vi "main.vi"() -> ()   [LabVIEW 2018]
uses:
  Ctrls/state.ctl
panel:
  out "Raw signal":u8[](graph)
  out "Output image":picture
  in  "Stop":bool
  in  "Save Image":bool
  in  "Image Name":string
  in  "Image upside down":bool
  out "Processing...":bool
  in  "Decode":bool
  in  "Input File":path
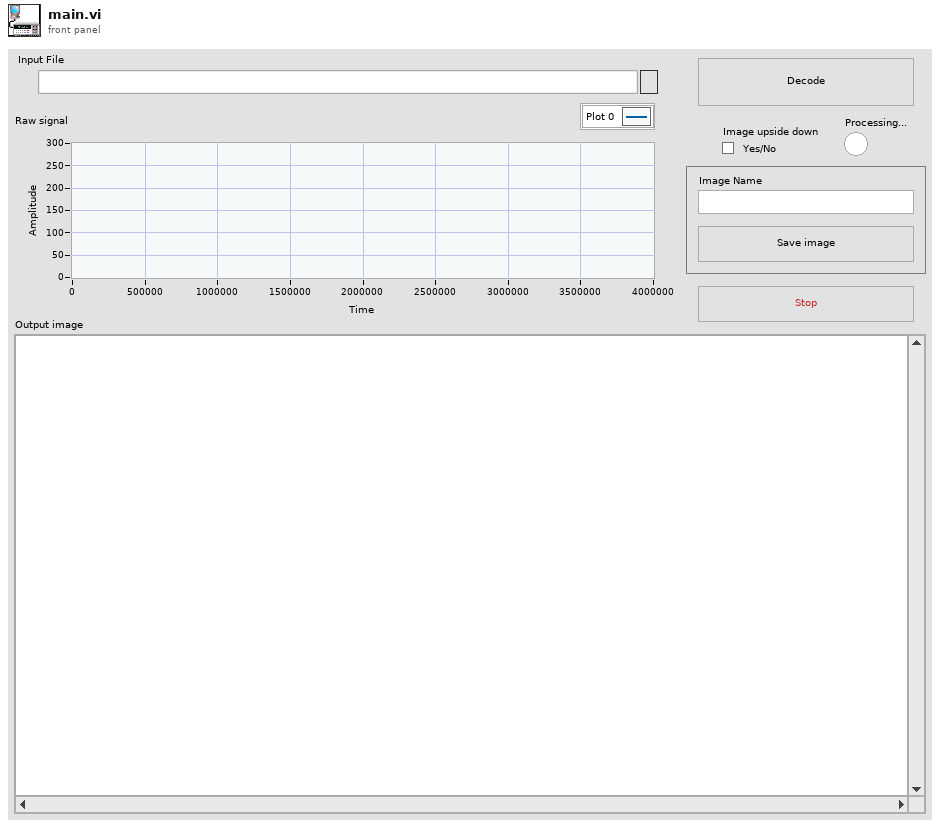
[diagram p1: front panel]
types:
  T1 = typedef "state.ctl" = enum16{"init", "decode", "quit", "UI", "save"}
  T2 = typedef "imagedata.ctl" = cluster{"image type":i32, "image depth":i32, "image":u8[], "mask":u8[], "colors":u32[], "Rectangle":cluster{"left":i16, "top":i16, "right":i16, "bottom":i16}}
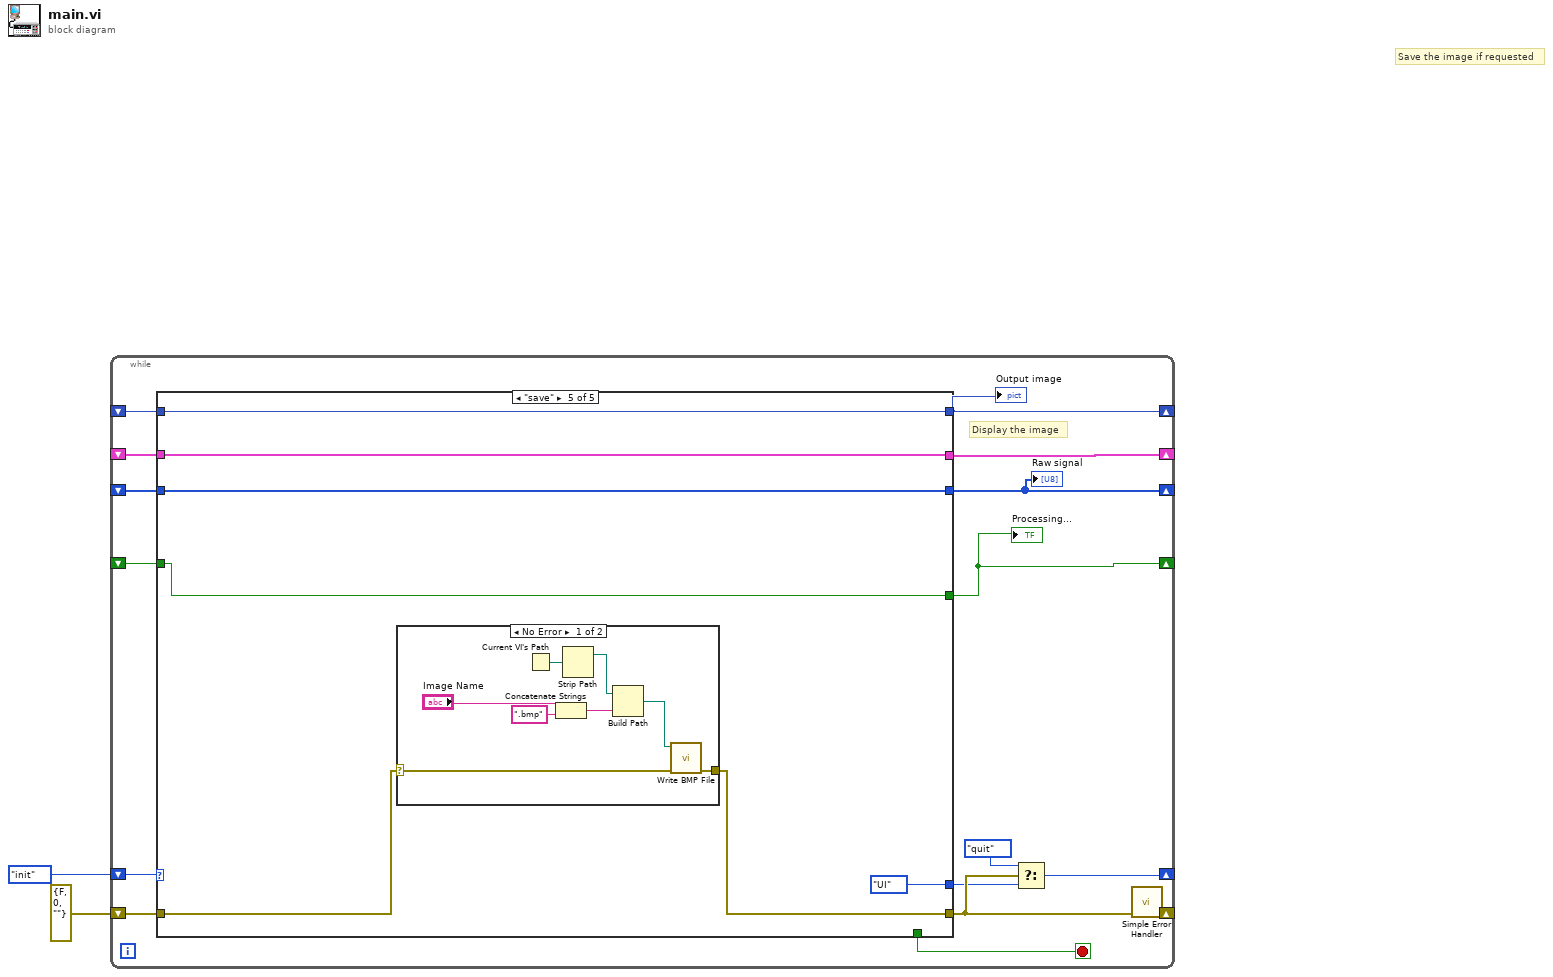
[diagram p0: block diagram]
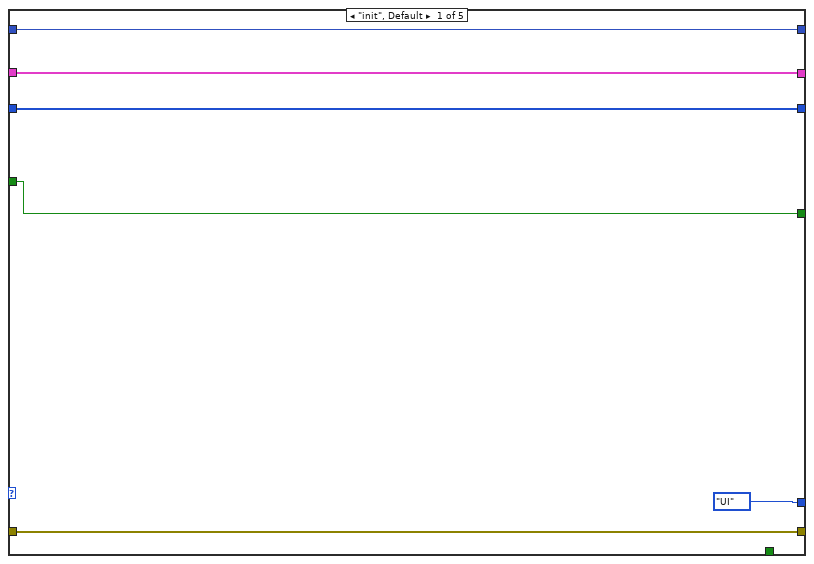
[diagram p2: hidden frame]
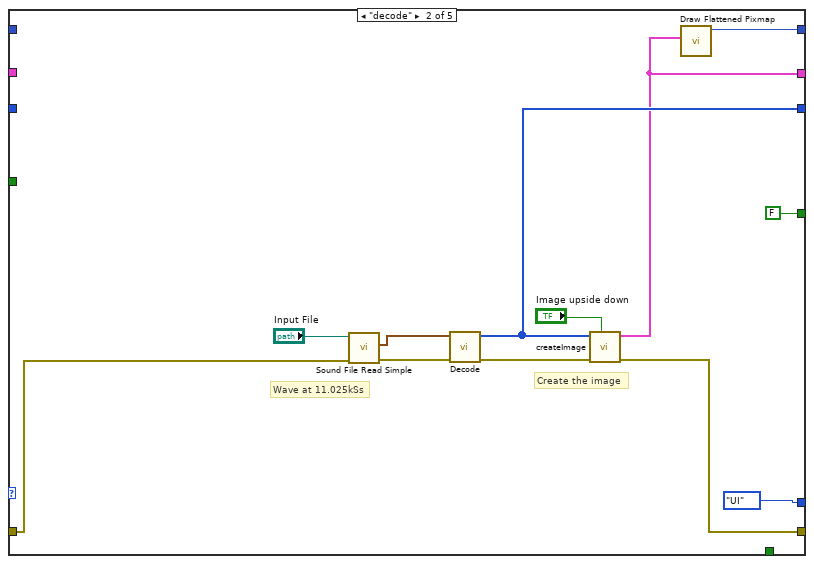
[diagram p3: hidden frame]
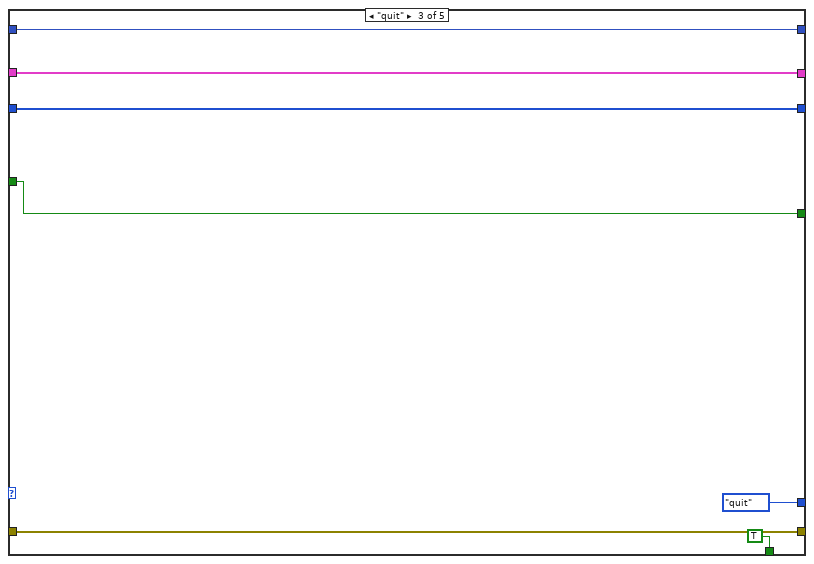
[diagram p4: hidden frame]
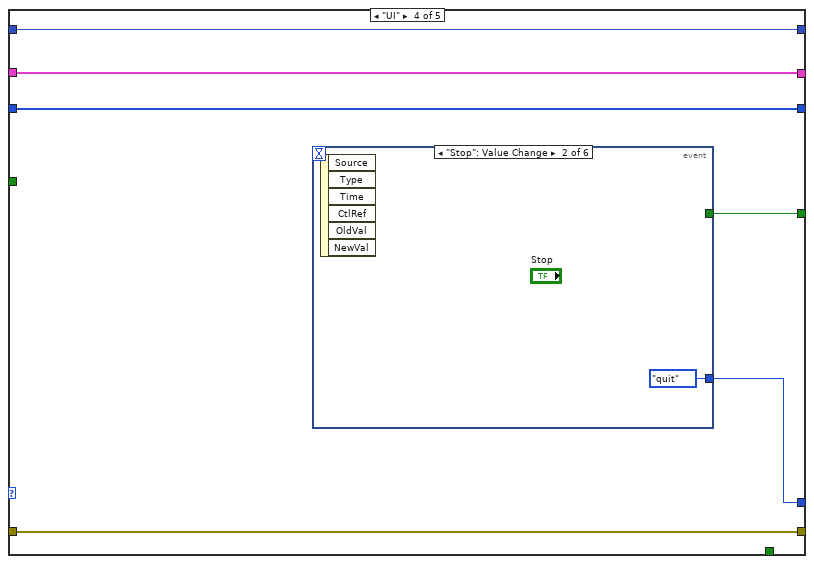
[diagram p5: hidden frame]
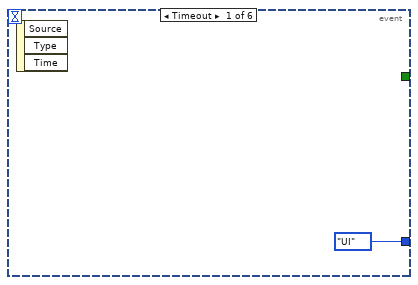
[diagram p6: hidden frame]
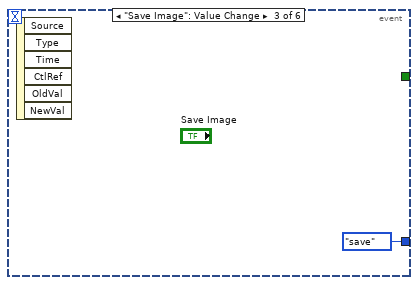
[diagram p7: hidden frame]
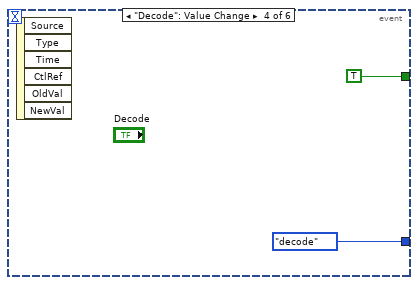
[diagram p8: hidden frame]
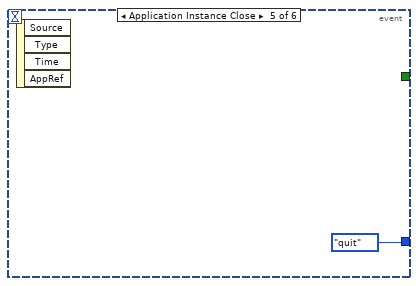
[diagram p9: hidden frame]
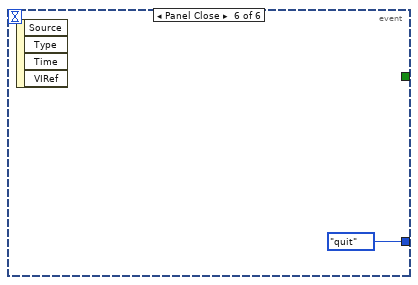
[diagram p10: hidden frame]
diagram:
  # "Save the image if requested"
  n1 = while {
    shift-right: [w13] -> _
    shift-left: state."init" -> [w18]
    shift-right: [w16] -> w1
    shift-left: errorcluster {"status"=FALSE, "code"=0, "source"=""} ("error constant") -> [w17]
    shift-right: [w4] -> _
    shift-left: _ -> [w9]
    shift-right: [w12] -> _
    shift-left: _ -> [w10]
    shift-right: [w5] -> _
    shift-left: _ -> [w11]
    shift-right: [w6] -> _
    shift-left: _ -> [w7]
    stop <- w8 stop-if-true
    # "Display the image"
    n2 = case shown="\"save\"" w18 {
      tunnel: w17 -> [w23 w31 w42 w49 w63]
      tunnel: [w23 w33 w42 w49 w62] -> w16
      tunnel: [state."UI" state."UI" state."quit" w48 state."UI"] -> w15
      tunnel: [w22 w30 w39 w47 w60] -> w4
      tunnel: [w21 w29 w40 w46 w59] -> w12
      tunnel: [w20 w28 w41 w45 w58] -> w5
      tunnel: w11 -> [w20 _ w41 w45 w58]
      tunnel: w10 -> [w21 _ w40 w46 w59]
      tunnel: w9 -> [w22 _ w39 w47 w60]
      tunnel: [_ _ TRUE _ _] -> w8
      tunnel: [w19 FALSE w37 w44 w57] -> w6
      tunnel: w7 -> [w19 _ w37 _ w57]
      frame "init", Default {
      }
      frame "decode" {
        # "Create the image"
        # "Wave at 11.025kSs"
        n3 = call <vilib>:"Sound File Read Simple.vi"("error in (no error)"=w31, "path"="Input File") -> ("error out"=w36:errorcluster, "data"=w35:waveform(dbl)[])  [unwired: 6 in, 2 out]
        n4 = call "Decode.vi"("error in (no error)"=w36, "data"=w35) -> ("error out"=w34:errorcluster, "Array"=w30:u8[])  [unwired: 8 in]
        n5 = call "createImage.vi"("Upside down"="Image upside down", "error in (no error)"=w34, "Array"=w30) -> ("error out"=w33:errorcluster, "image data"=w29:T2)  [unwired: 7 in]
        n6 = call <vilib>:"Draw Flattened Pixmap.vi"("image data"=w29) -> ("new picture"=w28:picture)  [unwired: 8 in]
      }
      frame "quit" {
      }
      frame "UI" {
        n7 = event shown="[1] \"Stop\": Value Change" {
          selector: _ -> [_ _ _ _ _ _]
          dyn-events: _ -> [_ _ _ _ _ _]
          timeout: _ -> [_ _ _ _ _ _]
          tunnel: [state."UI" state."quit" state."save" state."decode" state."quit" state."quit"] -> w48
          tunnel: [_ _ _ TRUE _ _] -> w44
          event Timeout {
            n8 = event-data() -> ()  [unwired: 1 in, 3 out]
          }
          event "Stop": Value Change {
            n9 = event-data() -> ()  [unwired: 1 in, 6 out]
          }
          event "Save Image": Value Change {
            n10 = event-data() -> ()  [unwired: 1 in, 6 out]
          }
          event "Decode": Value Change {
            n11 = event-data() -> ()  [unwired: 1 in, 6 out]
          }
          event Application Instance Close {
            n12 = event-data() -> ()  [unwired: 1 in, 4 out]
          }
          event Panel Close {
            n13 = event-data() -> ()  [unwired: 1 in, 4 out]
          }
        }
      }
      frame "save" {
        n14 = case shown="No Error" w63 {
          selector: w63 -> [w66 w72]
          tunnel: [w65 w72] -> w62
          frame No Error {
            n15 = Current VI's Path() -> (path=w69:path)
            n16 = Concatenate Strings("Image Name", ".bmp" ("string")) -> (w68:string)
            n17 = Strip Path(path=w69) -> (stripped path=w70:path)  [unwired: 1 out]
            n18 = Build Path(base path=w70, name or relative path=w68) -> (appended path=w71:path)
            n19 = call <vilib>:"Write BMP File.vi"("error in (no error)"=w66, "path to BMP file"=w71) -> ("error out"=w65:errorcluster)  [unwired: 8 in, 1 out]
          }
          frame Error {
          }
        }
      }
    }
    "Processing..." <- w6
    "Output image" <- w5
    "Raw signal" <- w4
    n20 = Select(t=state."quit", s=w16, f=w15) -> (s? t:f=w13:T1)
  }
  n21 = call <vilib>:"Simple Error Handler.vi"("error in (no error)"=w1) -> ()  [unwired: 4 in, 5 out]
